vi "Enter.vi"(8 "error in (no error)":errorcluster, 11 "MapSite in":refnum<class "MapSite.lvclass">) -> (0 "error out":errorcluster, 3 "MapSite out":refnum<class "MapSite.lvclass">)   [LabVIEW 2016, in "MapSite.lvclass"]
uses:
  MapSite.lvclass
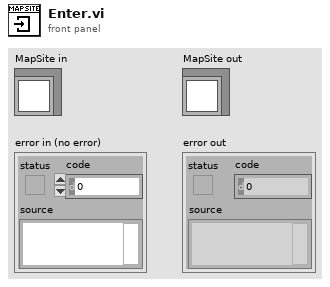
[diagram p1: front panel]
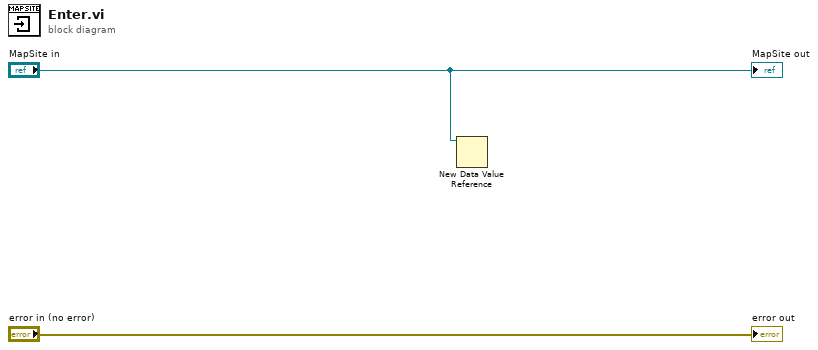
[diagram p0: block diagram]
diagram:
  n1 = New Data Value Reference(data value="MapSite in") -> ()  [unwired: 1 in, 2 out]
  "error out" <- "error in (no error)"
  "MapSite out" <- "MapSite in"
